vi "Detect Blocks.vi"(7 "client handle":T2, 8 "error in (no error)":errorcluster, 9 "Url":string, 10 "Image Dst":T1, 11 "Refnum in":T1) -> (0 "error out":errorcluster, 2 "Detected Image Out":T1, 3 "Camer Image out":T1)   [LabVIEW 2012]
uses:
  <vilib>/httpClient/ClientHandle.ctl
  <vilib>/vision/Image Controls.llb/IMAQ Image.ctl
  <vilib>/vision/NI_Vision_Development_Module.lvlib
  <vilib>/httpClient/LabVIEWHTTPClient.lvlib
panel:
  in  "Show image":bool
  out "Camera":T1(plugin-control)
  in  "Val Range":cluster{"Lower value":i32, "Upper value":i32}={"Lower value"=0, "Upper value"=179}
  in  "Sat Range":cluster{"Lower value":i32, "Upper value":i32}={"Lower value"=25, "Upper value"=200}
  in  "Hue Range":cluster{"Lower value":i32, "Upper value":i32}={"Lower value"=0, "Upper value"=200}
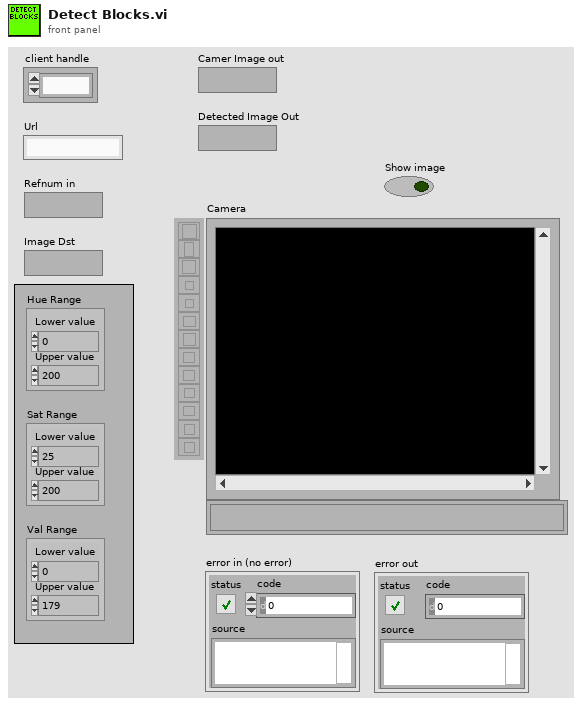
[diagram p1: front panel]
types:
  T1 = typedef "IMAQ Image.ctl" = refnum<image>
  T2 = typedef "LabVIEWHTTPClient.lvlib/ClientHandle.ctl" = refnum<k1>
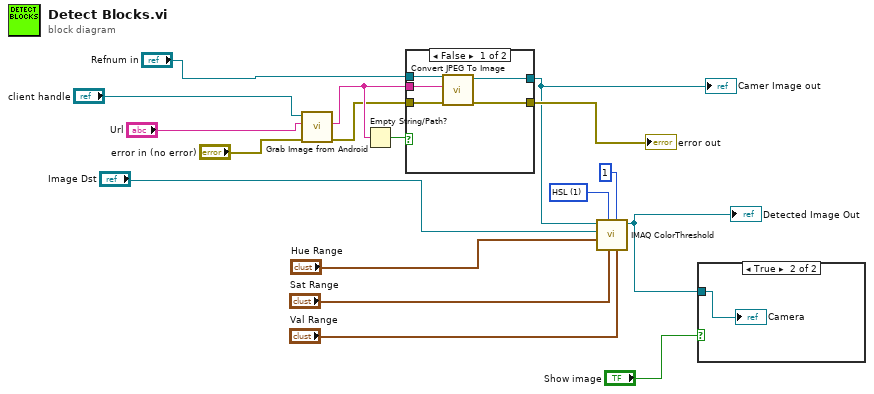
[diagram p0: block diagram]
diagram:
  w9 = u16 1 items=["RGB", "HSL", "HSV", "HSI"] ("Color Mode")
  n1 = call "Grab Image from Android.vi"("error in (no error)"="error in (no error)", "url"="Url", "client handle"="client handle") -> ("error out"=w7:errorcluster, "data out"=w17:string)  [unwired: 6 in, 1 out]
  n2 = Empty String/Path?(string/path=w17) -> (empty?=w6:bool)
  n3 = case shown="False" w6 {
    tunnel: "Refnum in" -> [w22 w23]
    tunnel: w7 -> [w21 w24]
    tunnel: [w20 w24] -> w4
    tunnel: [w19 w23] -> w2
    tunnel: w17 -> [w18 _]
    frame False {
      n4 = call "Convert JPEG To Image.vi"("error in"=w21, "Compressed Image"=w18, "Image In"=w22) -> ("error out"=w20:errorcluster, "Image Out"=w19:T1)  [unwired: 7 in]
    }
    frame True {
    }
  }
  "Camer Image out" <- w2
  "error out" <- w4
  n5 = call "IMAQ ColorThreshold"("Blue or Luma or Val or Inten Range"="Val Range", "Replace Value"=1, "Green or Sat Range"="Sat Range", "Color Mode"=w9, "Red or Hue Range"="Hue Range", "Image Dst"="Image Dst", "Image Src"=w2) -> ("Image Dst Out"=w1:T1)  [unwired: 3 in, 1 out]
  "Detected Image Out" <- w1
  n6 = case shown="True" "Show image" {
    tunnel: w1 -> [_ w25]
    frame False {
    }
    frame True {
      "Camera" <- w25
    }
  }
